vi "Remove Residue from Denominator (CDB).vi"(10 "Denominator":cdb[](array[numeric]) format="%#.6g", 11 "Numerator":cdb[](array[numeric]) format="%#.6g") -> (0 "error":i32, 2 "Denominator Out":cdb[](array[numeric]) format="%#.6g", 3 "Numerator Out":cdb[](array[numeric]) format="%#.6g")   [LabVIEW 2017, in "NI_AALPro.lvlib"]
doc: "Removes the residue from the denominator if the numerator equals zero. The data types you wire to the <B>Numerator</B> and <B>Denominator</B> inputs determine the polymorphic instance to use."
uses:
  NI_AALPro.lvlib
  Remove Zero Coefficients (CDB).vi
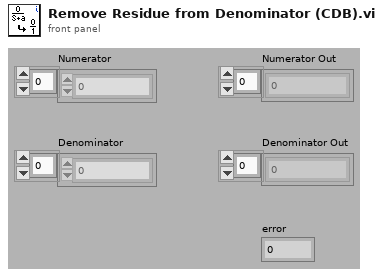
[diagram p1: front panel]
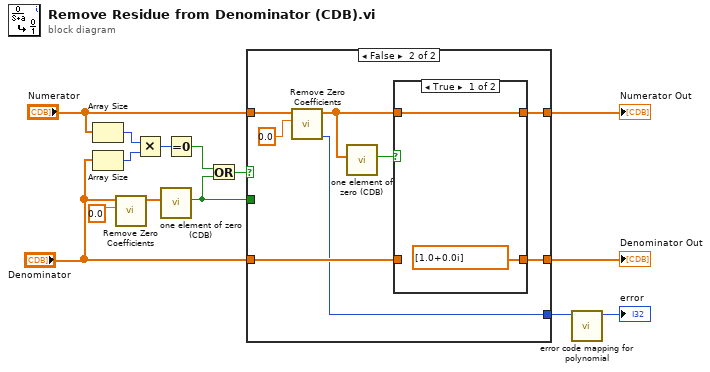
[diagram p0: block diagram]
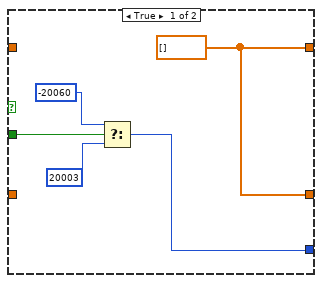
[diagram p2: hidden frame]
diagram:
  n1 = Array Size(array="Numerator") -> (size(s)=w11:i32)
  n2 = Array Size(array="Denominator") -> (size(s)=w10:i32)
  n3 = call-poly "Remove Zero Coefficients.vi"("threshold"=0.0, "P(x) In"="Denominator") -> ("P(x) Out"=w9:cdb[])  [unwired: 7 in, 2 out]
  n4 = Multiply(x=w11, y=w10) -> (x*y=w6:i32)
  n5 = call "one element of zero (CDB).vi"("Array in"=w9) -> ("equal [0]?"=w3:bool)  [unwired: 10 in]
  n6 = Equal To 0?(x=w6) -> (x = 0?=w5:bool)
  n7 = Or(x=w5, y=w3) -> (x .or. y?=w4:bool)
  n8 = case shown="False" w4 {
    tunnel: "Denominator" -> [_ w27]
    tunnel: [w19 w26] -> w14
    tunnel: [w19 w25] -> w13
    tunnel: "Numerator" -> [_ w24]
    tunnel: [w15 w20] -> w2
    tunnel: w3 -> [w18 _]
    frame True {
      w19 = cdb[] [] ("CDB")
      n9 = Select(t=-20060 ("divide by zero"), s=w18, f=20003 ("empty array")) -> (s? t:f=w15:i32)
    }
    frame False {
      n10 = call-poly "Remove Zero Coefficients.vi"("threshold"=0.0, "P(x) In"=w24) -> ("error"=w20:i32, "P(x) Out"=w21:cdb[])  [unwired: 7 in, 1 out]
      n11 = call "one element of zero (CDB).vi"("Array in"=w21) -> ("equal [0]?"=w22:bool)  [unwired: 10 in]
      n12 = case shown="True" w22 {
        tunnel: w21 -> [w29 w31]
        tunnel: w27 -> [_ w30]
        tunnel: [cdb[] [1.0+0.0i] ("denominator") w30] -> w25
        tunnel: [w29 w31] -> w26
        frame True {
        }
        frame False {
        }
      }
    }
  }
  "Denominator Out" <- w13
  "Numerator Out" <- w14
  n13 = call "error code mapping for polynomial.vi"("error in"=w2) -> ("error out"=→"error":i32)  [unwired: 10 in]
